vi "MB Read Registers.vi"(4 "Timeout":u32=2000, 8 "error in":errorcluster, 9 "MB status in":T1 {"MB update(s)" format="%.2g"; "ProCoDA Request"."PC update (s)" format="%.2f"; "ProCoDA Request"."# registers" min=1}, 10 "MB ID-Address":T5, 11 "VISA resource name":refnum<visa-resource-name>) -> (0 "error out":errorcluster, 1 "MB status out":T1 {"MB update(s)" format="%.2g"; "ProCoDA Request"."PC update (s)" format="%.2f"; "ProCoDA Request"."# registers" min=1}, 2 "Meter reading":sgl, 3 "VISA resource name out":refnum<visa-resource-name>, 5 "device ID out":u16)   [LabVIEW 2019]
doc: "The master uses this VI to read the slaves input registers. This corresponds to a public function code of 4 in the MODBUS protocol."
uses:
  MB status.ctl
  ProCoDA MB Request.ctl
  Read Write.ctl
  Modbus devices/byte swap.ctl
  MB ID-Address.ctl
  SerialParameters.ctl
  MB Modbus Command.ctl
panel:
  out "Exception Code":u8 format="%.0x"
  # "120 ms is too short for AccUView"
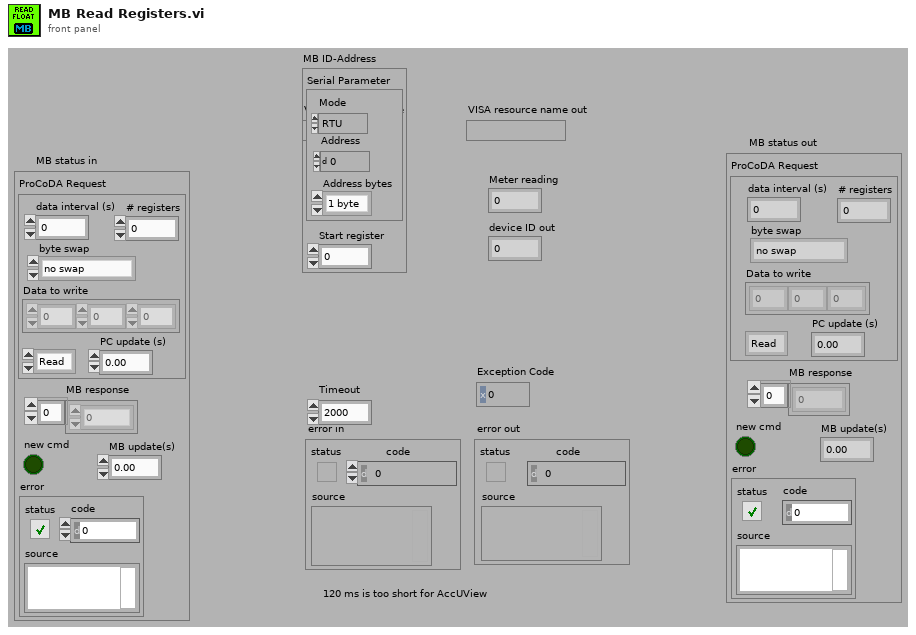
[diagram p1: front panel]
types:
  T1 = typedef "MB status.ctl" = cluster{"ProCoDA Request":T2, "MB response":dbl[], "new cmd":bool, "error":errorcluster, "MB update(s)":dbl}
  T2 = typedef "ProCoDA MB Request.ctl" = cluster{"# registers":u8, "Data to write":u16[], "data interval (s)":dbl, "command":T3, "PC update (s)":dbl, "byte swap":T4}
  T3 = typedef "Read Write.ctl" = enum16{"Read", "Write"}
  T4 = typedef "byte swap.ctl" = enum16{"no swap", "swap registers"}
  T5 = typedef "MB ID-Address.ctl" = cluster{"Serial Parameter":T6, "Start register":u16}
  T6 = typedef "SerialParameters.ctl" = cluster{"Mode":enum16{"RTU", "ASCII"}, "Address":u16, "Address bytes":enum16{"1 byte", "2 bytes"}}
  T7 = typedef "MB Modbus Command.ctl" = cluster{"Function Code":u8, "Starting Address":u16, "Quantity":u16, "Data":u16[], "Discrete":bool[]}
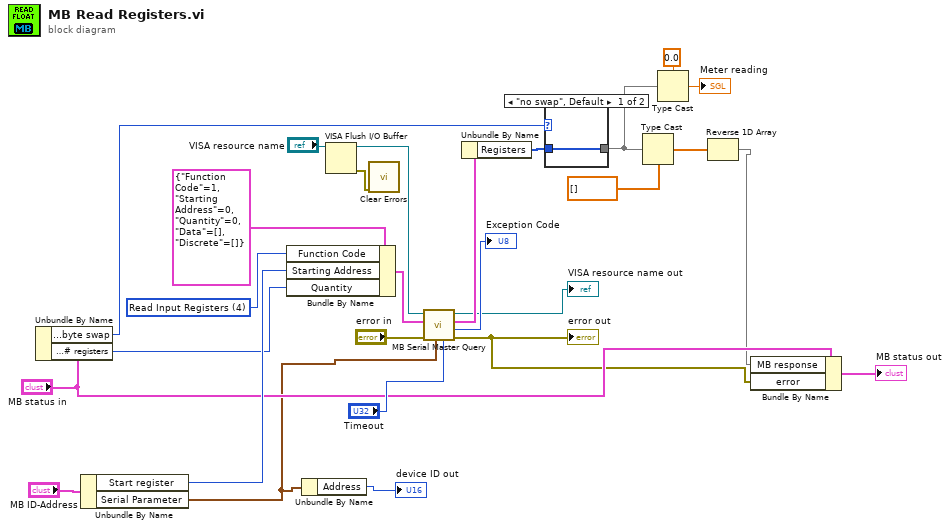
[diagram p0: block diagram]
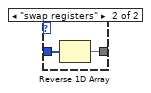
[diagram p2: hidden frame]
diagram:
  w25 = u8 4 items=["Read Coils"=1, "Read Discrete Inputs"=2, "Read Holding Registers"=3, "Read Input Registers"=4, "Write Single Coil"=5, "Write Single Register"=6, "Read Exception Status"=7, "Write Multiple Coils"=15, "Write Multiple Registers"=16] ("Function Code")
  n1 = Unbundle By Name("MB status in") -> ("ProCoDA Request.byte swap"=w1:T4, "ProCoDA Request.# registers"=w11:u8)
  n2 = Unbundle By Name("MB ID-Address") -> ("Start register"=w12:u16, "Serial Parameter"=w5:T6)
  n3 = Bundle By Name(cluster=T7 {"Function Code"=1, "Starting Address"=0, "Quantity"=0, "Data"=[], "Discrete"=[]} ("Modbus Command"), "Function Code"=w25, "Starting Address"=w12, "Quantity"=w11) -> (w26:T7)
  n4 = Unbundle By Name(w5) -> ("Address"=→"device ID out":u16)
  n5 = VISA Flush I/O Buffer(VISA resource name="VISA resource name") -> (VISA resource name out=w18:refnum<visa-resource-name>, error out=w14:errorcluster)  [unwired: 2 in]
  n6 = call <vilib>:"Clear Errors.vi"("error in (no error)"=w14) -> ()  [unwired: 5 in, 2 out]
  n7 = call "MB Serial Master Query.vi"("Timeout"="Timeout", "Serial Parameters"=w5, "error in (no error)"="error in", "Modbus Command"=w26, "VISA resource name"=w18) -> ("error out"=w6:errorcluster, "Exception Code"=→"Exception Code":u8, "Registers"=w21:cluster{"Registers":u16[], "Discrete":bool[]}, "VISA resource name out"=→"VISA resource name out":refnum<visa-resource-name>)  [unwired: 2 in, 1 out]
  "error out" <- w6
  n8 = Unbundle By Name(w21) -> ("Registers"=w3:u16[])
  n9 = case shown="\"no swap\", Default" w1 {
    tunnel: [w28 w30] -> w17
    tunnel: w3 -> [w28 w29]
    frame "no swap", Default {
    }
    frame "swap registers" {
      n10 = Reverse 1D Array(array=w29) -> (reversed array=w30:u16[])
    }
  }
  n11 = Type Cast(type=sgl[] [], x=w17) -> (*(type *) &x=w15:sgl[])
  n12 = Type Cast(type=sgl 0.0, x=w17) -> (*(type *) &x=→"Meter reading":sgl)
  n13 = Reverse 1D Array(array=w15) -> (reversed array=w7:sgl[])
  n14 = Bundle By Name(cluster="MB status in", "MB response"=w7, "error"=w6) -> (→"MB status out":T1)
